vi "Read Locals.vi"(9 "Diagram in":refnum<class "Diagram.lvclass">) -> (3 "Diagram out":refnum<class "Diagram.lvclass">, 4 "Locals":refnum<class "Local.lvclass">[](array[class]))   [LabVIEW 2014, in "Diagram.lvclass"]
uses:
  Diagram.lvclass
  Local/Local.lvclass
  Diagram.lvclass/Diagram.ctl
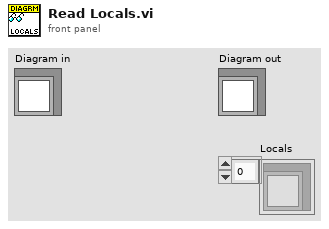
[diagram p1: front panel]
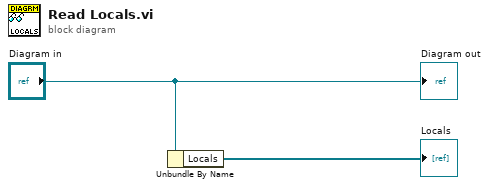
[diagram p0: block diagram]
diagram:
  n1 = Unbundle By Name("Diagram in") -> ("Locals"=→"Locals":refnum<class "Local.lvclass">[])
  "Diagram out" <- "Diagram in"
